vi "AlliGator Compute Lifetime Variance Map (Core).vi"(6 "Build New Maps":bool, 7 "Function Parameters":T1={"Function"=enum."Single-Exponential", "Amplitude"=0.0, "Exponent/Scale"=0.0, "Baseline"=0.0, "Residuals SDV"=0.0, "Minimum CL (%)"=1.0, "Analysis Type"=enum."Reference", "Bootstrap SDV x Scale Factor"=1.0, "Residuals SDV x Scale Factor"=1.0, "Low CL Percentile to Reject (%)"=1.0} {"Low CL Percentile to Reject (%)" min=0.0 max=100.0; "Residuals SDV x Scale Factor" min=0.0 max=100.0; "Bootstrap SDV x Scale Factor" min=0.0 max=100.0; "Minimum CL (%)" min=1.0}, 8 "error in (no error)":errorcluster, 11 "Lifetime Variance Data Array":T3[](array[typedef])) -> (0 "error out":errorcluster, 1 "CV Bootstrap SDV Test kappa x SDV":dbl, 2 "CV Residual Test kappa x SDV":dbl, 3 "Maps Data":dbl[][](array[numeric]))   [LabVIEW 2021, in "AlliGator Decay Fit Parameter Map.lvlib"]
uses:
  Decay Fit Parameter Map/AlliGator Decay Fit Parameter Map.lvlib
  Camera Noise Influence on Lifetime/Lifetime Variance Data.ctl
  Decay Fit Parameter Map/AlliGator Function Parameters.ctl
  Decay Fit Parameter Map/AlliGator CV(tau) Model Function.ctl
  Decay Fit Parameter Map/AlliGator Lifetime Variance Statistical Test.ctl
  <vilib>/gmath/statdist.llb/F CDF.vi
  <vilib>/gmath/statdist.llb/Normal CDF.vi
  <vilib>/gmath/statdist.llb/Normal Inverse CDF.vi
  <userlib>/_OpenG.lib/array/array.llb/Index 1D Array Elements (DBL)__ogtk.vi
  Error/Error.lvlib
  <vilib>/gmath/NI_Gmath.lvlib
  Arrays/Arrays.lvlib
  <userlib>/_OpenG.lib/array/array.llb/openg_array.lvlib
  Lifetime & Other Parameters/AlliGator Lifetime & Other Parameters.lvlib
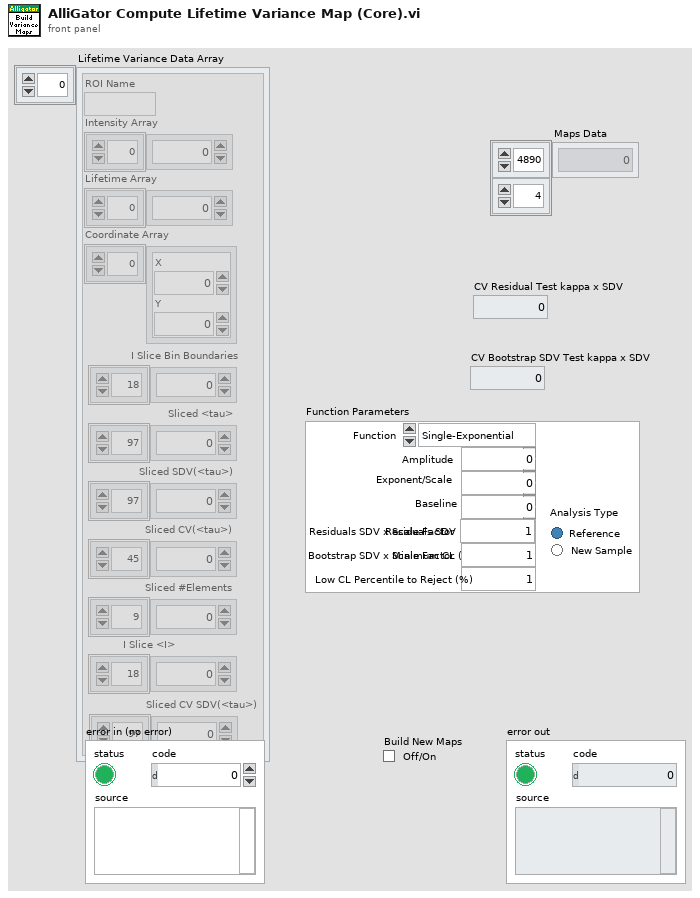
[diagram p1: front panel]
types:
  T1 = typedef "AlliGator Decay Fit Parameter Map.lvlib/AlliGator Function Parameters.ctl" = cluster{"Function":T2, "Amplitude":dbl, "Exponent/Scale":dbl, "Baseline":dbl, "Residuals SDV":dbl, "Minimum CL (%)":dbl, "Analysis Type":enum32{"Reference", "New Sample"}, "Bootstrap SDV x Scale Factor":dbl, "Residuals SDV x Scale Factor":dbl, "Low CL Percentile to Reject (%)":dbl}
  T2 = typedef "AlliGator Lifetime & Other Parameters.lvlib/AlliGator CV(tau) Model Function.ctl" = enum16{"Single-Exponential", "Power Law"}
  T3 = typedef "AlliGator Decay Fit Parameter Map.lvlib/Lifetime Variance Data.ctl" = cluster{"ROI Name":string, "Intensity Array":sgl[], "Lifetime Array":dbl[], "Coordinate Array":cluster{"X":i32, "Y":i32}[], "I Slice Bin Boundaries":dbl[], "Sliced <tau>":dbl[], "Sliced SDV(<tau>)":dbl[], "Sliced CV(<tau>)":dbl[], "Sliced #Elements":i32[], "I Slice <I>":dbl[], "Sliced CV SDV(<tau>)":dbl[]}
  T4 = typedef "AlliGator Decay Fit Parameter Map.lvlib/AlliGator Lifetime Variance Statistical Test.ctl" = enum16{"CV Approximate F-test", "Variance F-test", "CV Residuals test", "CV Bootstrap SDV Test"}
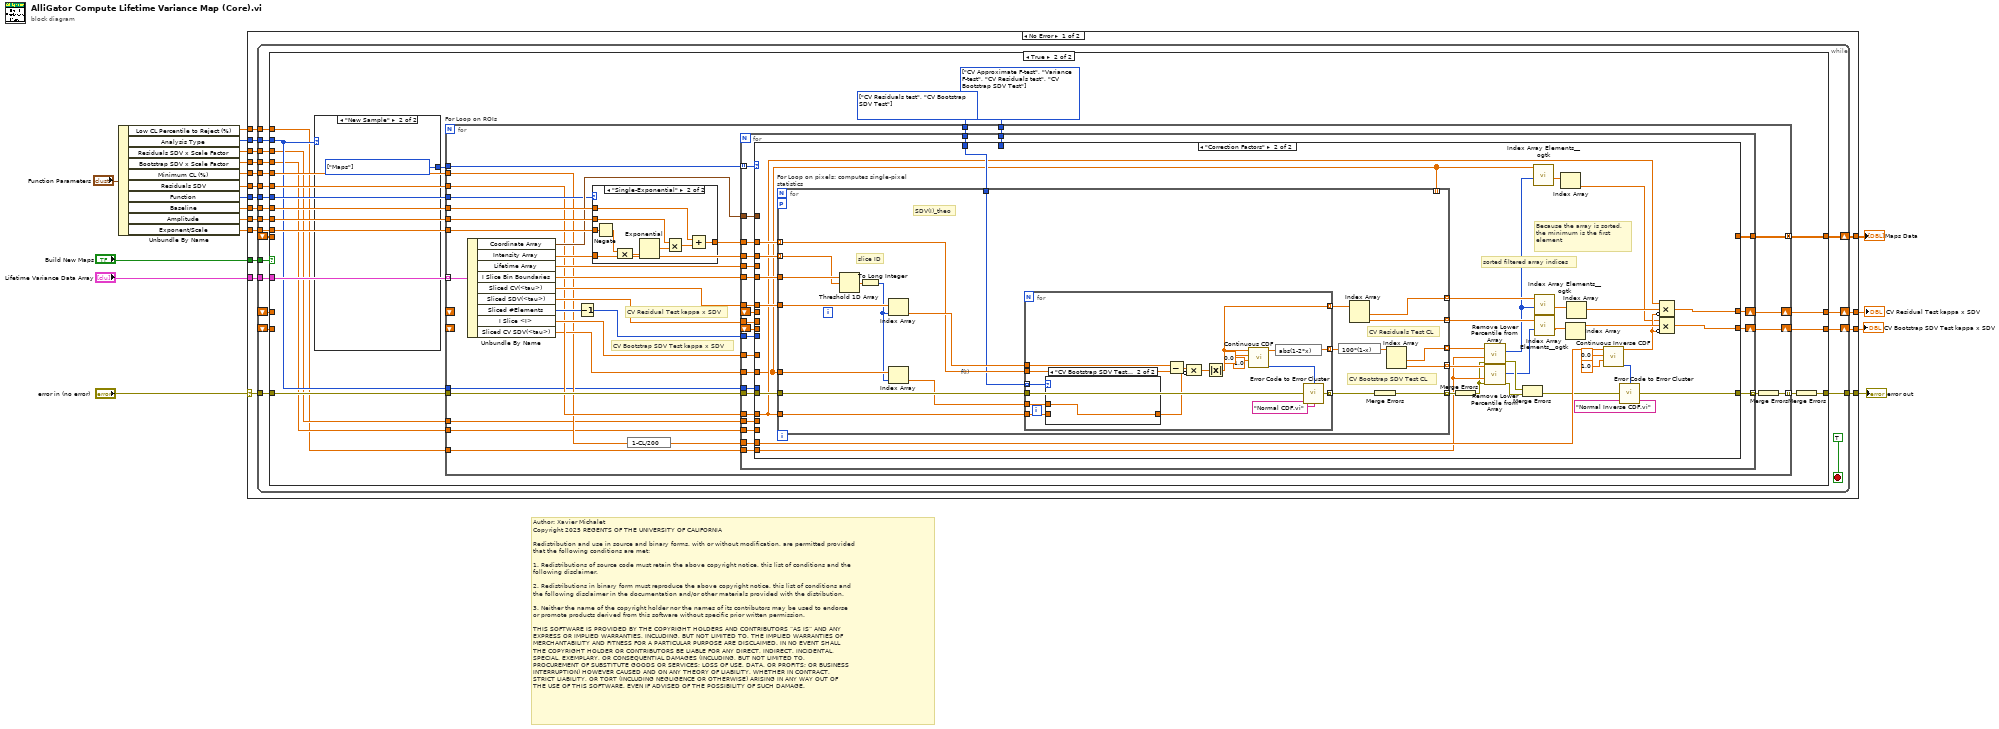
[diagram p0: block diagram]
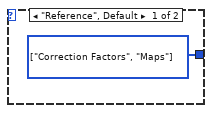
[diagram p3: hidden frame]
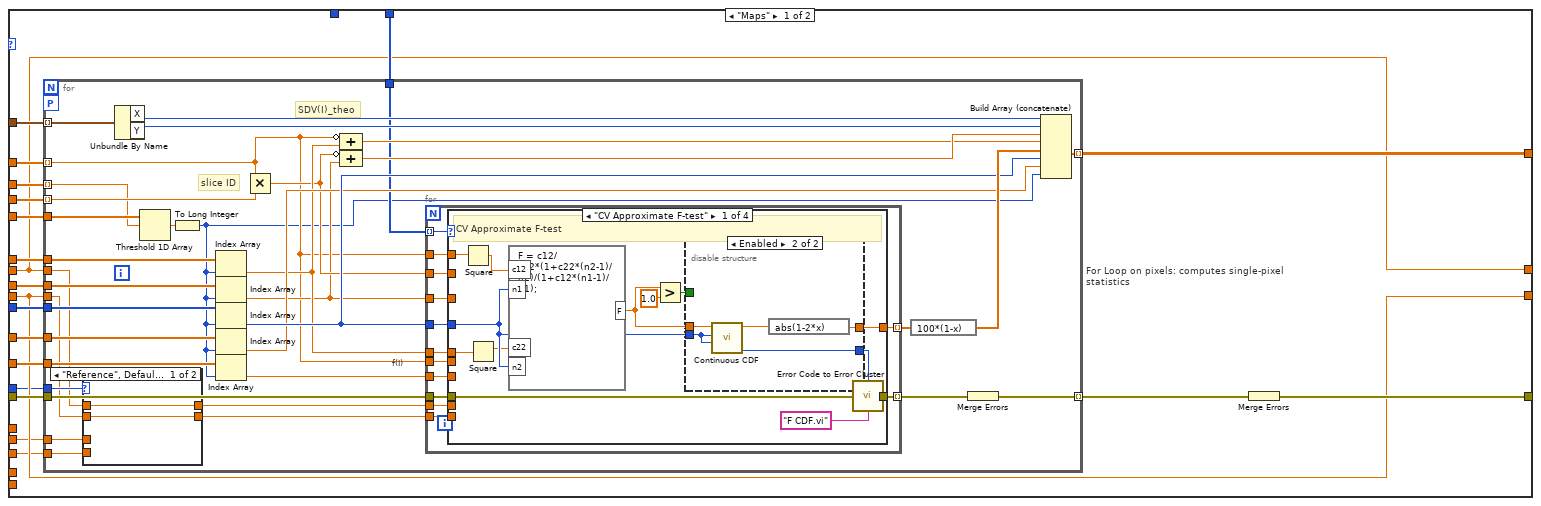
[diagram p4: hidden frame]
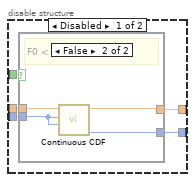
[diagram p6: hidden frame]
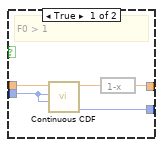
[diagram p7: hidden frame]
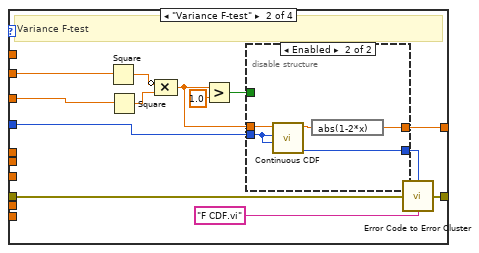
[diagram p8: hidden frame]
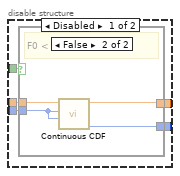
[diagram p9: hidden frame]
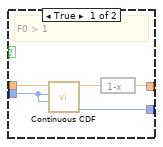
[diagram p10: hidden frame]
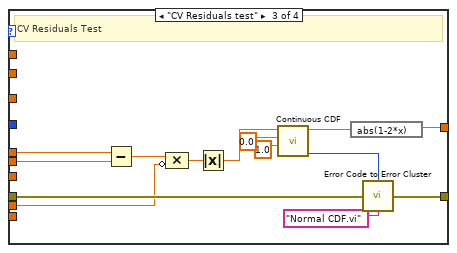
[diagram p11: hidden frame]
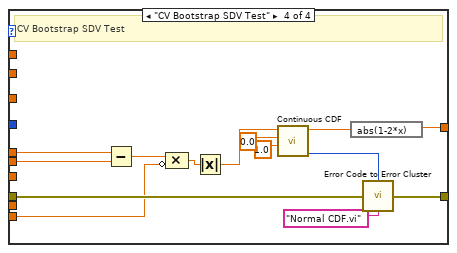
[diagram p12: hidden frame]
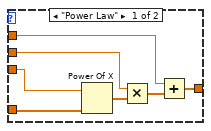
[diagram p14: hidden frame]
diagram:
  # "Author: Xavier Michalet\nCopyright 2025 REGENTS OF THE UNIVERSITY OF CALIFORNIA\n\nRedistribution and use in source and binary forms, with or without modification, are permitted provided\nthat the following conditions are met:\n\n1. Redistributions of source code must retain the above copyright notice, this list of conditions and the\nfollowing disclaimer.\n\n2. Redistributions in binary form must reproduce the above copyright notice, this list of conditions and\nthe following disclaimer in the documentation and/or other materials provided with the distribution.\n\n3. Neither the name of the copyright holder nor the names of its contributors may be used to endorse \nor promote products derived from this software without specific prior written permission.\n\nTHIS SOFTWARE IS PROVIDED BY THE COPYRIGHT HOLDERS AND CONTRIBUTORS “AS IS” AND ANY \nEXPRESS OR IMPLIED WARRANTIES, INCLUDING, BUT NOT LIMITED TO, THE IMPLIED WARRANTIES OF\nMERCHANTABILITY AND FITNESS FOR A PARTICULAR PURPOSE ARE DISCLAIMED. IN NO EVENT SHALL\nTHE COPYRIGHT HOLDER OR CONTRIBUTORS BE LIABLE FOR ANY DIRECT, INDIRECT, INCIDENTAL, \nSPECIAL, EXEMPLARY, OR CONSEQUENTIAL DAMAGES (INCLUDING, BUT NOT LIMITED TO, \nPROCUREMENT OF SUBSTITUTE GOODS OR SERVICES; LOSS OF USE, DATA, OR PROFITS; OR BUSINESS\nINTERRUPTION) HOWEVER CAUSED AND ON ANY THEORY OF LIABILITY, WHETHER IN CONTRACT, \nSTRICT LIABILITY, OR TORT (INCLUDING NEGLIGENCE OR OTHERWISE) ARISING IN ANY WAY OUT OF\nTHE USE OF THIS SOFTWARE, EVEN IF ADVISED OF THE POSSIBILITY OF SUCH DAMAGE."
  n1 = Unbundle By Name("Function Parameters") -> ("Low CL Percentile to Reject (%)"=w1:dbl, "Analysis Type"=w4:enum32{"Reference", "New Sample"}, "Residuals SDV x Scale Factor"=w3:dbl, "Bootstrap SDV x Scale Factor"=w2:dbl, "Minimum CL (%)"=w7:dbl, "Residuals SDV"=w8:dbl, "Function"=w9:T2, "Baseline"=w14:dbl, "Amplitude"=w15:dbl, "Exponent/Scale"=w16:dbl)
  n2 = case shown="No Error" "error in (no error)" {
    selector: "error in (no error)" -> [w28 w397]
    tunnel: "Lifetime Variance Data Array" -> [w35 _]
    tunnel: w16 -> [w34 _]
    tunnel: w15 -> [w33 _]
    tunnel: w14 -> [w32 _]
    tunnel: [w31 _] -> w13
    tunnel: "Build New Maps" -> [w30 _]
    tunnel: [w29 w397] -> w10
    tunnel: w9 -> [w27 _]
    tunnel: w8 -> [w26 _]
    tunnel: w7 -> [w25 _]
    tunnel: [w24 _] -> w6
    tunnel: [w23 _] -> w5
    tunnel: w4 -> [w22 _]
    tunnel: w3 -> [w21 _]
    tunnel: w2 -> [w20 _]
    tunnel: w1 -> [w19 _]
    frame No Error {
      n3 = while {
        tunnel: w35 -> [w56]
        tunnel: w34 -> [w55]
        tunnel: w33 -> [w54]
        tunnel: w32 -> [w53]
        tunnel: w30 -> [w51]
        shift-right: [w52] -> w31
        shift-left: _ -> [w49]
        tunnel: [w48] -> w29
        tunnel: w28 -> [w47]
        tunnel: w27 -> [w46]
        tunnel: w26 -> [w45]
        tunnel: w25 -> [w44]
        shift-right: [w43] -> w24
        shift-left: _ -> [w41]
        shift-right: [w42] -> w23
        shift-left: _ -> [w40]
        tunnel: w22 -> [w39]
        tunnel: w21 -> [w38]
        tunnel: w20 -> [w37]
        tunnel: w19 -> [w36]
        stop <- TRUE stop-if-true
        n4 = case shown="True" w51 {
          tunnel: w56 -> [_ w80]
          tunnel: w55 -> [_ w79]
          tunnel: w54 -> [_ w78]
          tunnel: w53 -> [_ w77]
          tunnel: [w60 w76] -> w52
          tunnel: w49 -> [w60 _]
          tunnel: [w59 w74] -> w48
          tunnel: w47 -> [w59 w73]
          tunnel: w46 -> [_ w72]
          tunnel: w45 -> [_ w71]
          tunnel: w44 -> [_ w69]
          tunnel: [w58 w67] -> w43
          tunnel: [w57 w66] -> w42
          tunnel: w41 -> [w58 _]
          tunnel: w40 -> [w57 _]
          tunnel: w39 -> [_ w64]
          tunnel: w38 -> [_ w63]
          tunnel: w37 -> [_ w62]
          tunnel: w36 -> [_ w61]
          frame False {
          }
          frame True {
            w68 = T4[] [enum."CV Residuals test", enum."CV Bootstrap SDV Test"] items=["CV Approximate F-test", "Variance F-test", "CV Residuals test", "CV Bootstrap SDV Test"]
            w70 = T4[] [enum."CV Approximate F-test", enum."Variance F-test", enum."CV Residuals test", enum."CV Bootstrap SDV Test"] items=["CV Approximate F-test", "Variance F-test", "CV Residuals test", "CV Bootstrap SDV Test"]
            n5 = case shown="\"New Sample\"" w64 {
              tunnel: [w81 w82] -> w65
              frame "Reference", Default {
                w81 = enum16{"Correction Factors", "Maps"}[] [enum."Correction Factors", enum."Maps"] items=["Correction Factors", "Maps"]
              }
              frame "New Sample" {
                w82 = enum16{"Correction Factors", "Maps"}[] [enum."Maps"] items=["Correction Factors", "Maps"]
              }
            }
            n6 = for "For Loop on ROIs" {
              tunnel: w80 -> [w114] mode=indexing
              tunnel: w79 -> [w113]
              tunnel: w78 -> [w112]
              tunnel: w77 -> [w111]
              tunnel: [w101] -> w76 mode=concatenating
              tunnel: [w99] -> w75 mode=indexing
              tunnel: w73 -> [w98]
              tunnel: w72 -> [w96]
              tunnel: w71 -> [w95]
              tunnel: w70 -> [w94]
              tunnel: w69 -> [w91]
              tunnel: w65 -> [w92]
              tunnel: w68 -> [w89]
              shift-right: [w88] -> w67
              shift-left: _ -> [_]
              shift-right: [w87] -> w66
              shift-left: _ -> [_]
              tunnel: w64 -> [w86]
              tunnel: w63 -> [w85]
              tunnel: w62 -> [w84]
              tunnel: w61 -> [w83]
              # "CV Bootstrap SDV Test kappa x SDV"
              # "CV Residual Test kappa x SDV"
              n7 = Unbundle By Name(w114) -> ("Coordinate Array"=w105:cluster{"X":i32, "Y":i32}[], "Intensity Array"=w104:sgl[], "Lifetime Array"=w110:dbl[], "I Slice Bin Boundaries"=w109:dbl[], "Sliced CV(<tau>)"=w108:dbl[], "Sliced SDV(<tau>)"=w106:dbl[], "Sliced #Elements"=w103:i32[], "I Slice <I>"=w97:dbl[], "Sliced CV SDV(<tau>)"=w93:dbl[])
              n8 = Decrement(x=w103) -> (x-1=w102:i32[])
              n9 = case shown="\"Single-Exponential\"" w96 {
                tunnel: w113 -> [w387 w389]
                tunnel: w112 -> [w385 w395]
                tunnel: w111 -> [w383 w393]
                tunnel: [w382 w392] -> w107
                tunnel: w104 -> [w381 w391]
                frame "Power Law" {
                  n10 = Power Of X(1:w381, 2:w387) -> (0:w386:dbl[])
                  n11 = Multiply(x=w385, y=w386) -> (x*y=w384:dbl[])
                  n12 = Add(x=w383, y=w384) -> (x+y=w382:dbl[])
                }
                frame "Single-Exponential" {
                  n13 = Negate(x=w389) -> (-x=w388:dbl)
                  n14 = Compound Arithmetic op=MULTIPLY(w388, w391) -> (w390:dbl[])
                  n15 = Exponential(1:w390) -> (0:w396:dbl[])
                  n16 = Multiply(x=w395, y=w396) -> (x*y=w394:dbl[])
                  n17 = Add(x=w393, y=w394) -> (x+y=w392:dbl[])
                }
              }
              n18 = expression code="1-CL/200"(w91) -> (w90:dbl)
              n19 = for {
                tunnel: w110 -> [w140]
                tunnel: w109 -> [w139]
                tunnel: w108 -> [w138]
                tunnel: w107 -> [w137]
                tunnel: w106 -> [w136]
                tunnel: w105 -> [w135]
                tunnel: w104 -> [w134]
                tunnel: w102 -> [w133]
                tunnel: [w132] -> w101
                tunnel: [w131] -> w100 mode=indexing
                tunnel: w98 -> [w130]
                tunnel: w97 -> [w129]
                tunnel: w95 -> [w128]
                tunnel: w94 -> [w127]
                tunnel: w93 -> [w126]
                tunnel: w90 -> [w125]
                tunnel: w92 -> [w124] mode=indexing
                shift-right: [w123] -> w88
                shift-left: _ -> [w121]
                shift-right: [w122] -> w87
                shift-left: _ -> [w120]
                tunnel: w89 -> [w119]
                tunnel: w86 -> [w118]
                tunnel: w85 -> [w117]
                tunnel: w84 -> [w116]
                tunnel: w83 -> [w115]
                n20 = case shown="\"Correction Factors\"" w124 {
                  tunnel: w140 -> [w160 _]
                  tunnel: w139 -> [w159 w340]
                  tunnel: w138 -> [w158 w339]
                  tunnel: w137 -> [w157 w338]
                  tunnel: w136 -> [w156 _]
                  tunnel: w135 -> [w155 _]
                  tunnel: w134 -> [w154 w337]
                  tunnel: w133 -> [w153 _]
                  tunnel: [w152 _] -> w132
                  tunnel: [w146 w328] -> w131
                  tunnel: w130 -> [w150 w335]
                  tunnel: w129 -> [w149 _]
                  tunnel: w128 -> [_ w310]
                  tunnel: w127 -> [w148 _]
                  tunnel: w126 -> [w147 w309]
                  tunnel: w125 -> [_ w325]
                  tunnel: [w145 w327] -> w123
                  tunnel: [w144 w326] -> w122
                  tunnel: w121 -> [w145 _]
                  tunnel: w120 -> [w144 _]
                  tunnel: w119 -> [_ w323]
                  tunnel: w118 -> [w143 _]
                  tunnel: w117 -> [w142 _]
                  tunnel: w116 -> [w141 _]
                  tunnel: w115 -> [_ w320]
                  frame "Maps" {
                    n21 = for "For Loop on pixels: computes single-pixel statistics" {
                      tunnel: w160 -> [w193] mode=indexing
                      tunnel: w159 -> [w196]
                      tunnel: w158 -> [w195]
                      tunnel: w157 -> [w172] mode=indexing
                      tunnel: w156 -> [w194]
                      tunnel: w155 -> [w192] mode=indexing
                      tunnel: w154 -> [w191] mode=indexing
                      tunnel: w153 -> [w186]
                      tunnel: [w183] -> w152 mode=indexing
                      tunnel: [w177] -> w151 mode=indexing
                      tunnel: w150 -> [w181]
                      tunnel: w149 -> [w180]
                      tunnel: w148 -> [w173]
                      tunnel: w147 -> [w171]
                      workers-P: _ -> [_]
                      tunnel: w145 -> [w166]
                      tunnel: w144 -> [w165]
                      tunnel: w143 -> [w167]
                      tunnel: w142 -> [w162]
                      tunnel: w141 -> [w161]
                      # "f(I)"
                      # "slice ID"
                      # "SDV(I)_theo"
                      n22 = case shown="\"Reference\", Default" w167 {
                        tunnel: w166 -> [w198 _]
                        tunnel: w165 -> [w197 _]
                        tunnel: [w198 w200] -> w164
                        tunnel: [w197 w199] -> w163
                        tunnel: w162 -> [_ w200]
                        tunnel: w161 -> [_ w199]
                        frame "Reference", Default {
                        }
                        frame "New Sample" {
                        }
                      }
                      n23 = Unbundle By Name(w192) -> ("X"=w190:i32, "Y"=w189:i32)
                      n24 = Threshold 1D Array(2:w191, 3:w196) -> (0:w170:dbl)  [unwired: 1 in]
                      n25 = To Long Integer(number=w170) -> (32bit integer=w168:i32)
                      n26 = Index Array(array=w195, index=w168) -> (element=w176:dbl)
                      n27 = Index Array(array=w194, index=w168) -> (element=w174:dbl)
                      n28 = Index Array(array=w186, index=w168) -> (element=w179:i32)
                      n29 = Index Array(array=w180, index=w168) -> (element=w178:dbl)
                      n30 = Index Array(array=w171, index=w168) -> (element=w169:dbl)
                      n31 = Multiply(x=w172, y=w193) -> (x*y=w175:dbl)
                      n32 = Compound Arithmetic op=ADD(invert w172, w176) -> (w187:dbl)
                      n33 = Compound Arithmetic op=ADD(invert w175, w174) -> (w188:dbl)
                      n34 = for {
                        tunnel: w179 -> [w210]
                        tunnel: w173 -> [w209] mode=indexing
                        tunnel: [w213] -> w185 mode=indexing
                        tunnel: w181 -> [w211]
                        tunnel: [w212] -> w182 mode=indexing
                        tunnel: w172 -> [w208]
                        tunnel: w176 -> [w207]
                        tunnel: w175 -> [w206]
                        tunnel: w174 -> [w205]
                        tunnel: w172 -> [w204]
                        tunnel: w169 -> [w203]
                        tunnel: w164 -> [w202]
                        tunnel: w163 -> [w201]
                        n35 = case shown="\"CV Approximate F-test\"" w209 {
                          tunnel: [w226 w258 w291 w305] -> w213
                          tunnel: [w225 w257 w290 w304] -> w212
                          tunnel: w211 -> [w222 w254 w287 w301]
                          tunnel: w210 -> [w216 w253 _ _]
                          tunnel: w208 -> [_ _ w284 w298]
                          tunnel: w207 -> [w218 _ w285 w299]
                          tunnel: w206 -> [_ w250 _ _]
                          tunnel: w205 -> [_ w249 _ _]
                          tunnel: w204 -> [w219 _ _ _]
                          tunnel: w203 -> [_ _ _ _]
                          tunnel: w202 -> [_ _ w278 _]
                          tunnel: w201 -> [_ _ _ w292]
                          frame "CV Approximate F-test" {
                            # "CV Approximate F-test"
                            n36 = Square(x=w219) -> (x^2=w217:dbl)
                            n37 = Square(x=w218) -> (x^2=w215:dbl)
                            n38 = formula code="F = c12/c22*(1+c22*(n2-1)/n2)/(1+c12*(n1-1)/n1);"("c12"=w217, "c22"=w215, "n1"=w216, "n2"=w216) -> ("F"=w214:dbl)
                            n39 = Greater?(x=w214, y=1.0) -> (0:w220:bool)
                            n40 = disable-structure shown="Enabled" {
                              disable-tunnel: [w231 w241] -> w226
                              disable-tunnel: [w230 w245] -> w224
                              disable-tunnel: w216 -> [w229 w244]
                              disable-tunnel: w214 -> [w228 w243]
                              disable-tunnel: w220 -> [w227 _]
                              frame Disabled {
                                n41 = case shown="False" w227 {
                                tunnel: w228 -> [w236 w240]
                                tunnel: [w232 w237] -> w231
                                tunnel: [w235 w239] -> w230
                                tunnel: w229 -> [w234 w238]
                                frame True {
                                # "F0 > 1"
                                n42 = call-poly <vilib>:"Continuous CDF.vi"("k2"=w234, "k1"=w234, "x"=w236) -> ("error"=w235:i32, "cdf(x)"=w233:dbl)  [unwired: 7 in]
                                n43 = expression code="1-x"(w233) -> (w232:dbl)
                                }
                                frame False {
                                # "F0 < 1"
                                n44 = call-poly <vilib>:"Continuous CDF.vi"("k2"=w238, "k1"=w238, "x"=w240) -> ("error"=w239:i32, "cdf(x)"=w237:dbl)  [unwired: 7 in]
                                }
                                }
                              }
                              frame Enabled {
                                n45 = call-poly <vilib>:"Continuous CDF.vi"("k2"=w244, "k1"=w244, "x"=w243) -> ("error"=w245:i32, "cdf(x)"=w242:dbl)  [unwired: 7 in]
                                n46 = expression code="abs(1-2*x)"(w242) -> (w241:dbl)
                              }
                            }
                            n47 = call "Error Code to Error Cluster.vi"("Error Code"=w224, "Error Source"="F CDF.vi", "Error In"=w222) -> ("Error Out"=w225:errorcluster)  [unwired: 12 in]
                          }
                          frame "Variance F-test" {
                            # "Variance F-test"
                            n48 = Square(x=w250) -> (x^2=w248:dbl)
                            n49 = Square(x=w249) -> (x^2=w251:dbl)
                            n50 = Compound Arithmetic op=MULTIPLY(invert w248, w251) -> (w247:dbl)
                            n51 = Greater?(x=w247, y=1.0) -> (0:w246:bool)
                            n52 = disable-structure shown="Enabled" {
                              disable-tunnel: [w263 w273] -> w258
                              disable-tunnel: [w262 w277] -> w256
                              disable-tunnel: w253 -> [w261 w276]
                              disable-tunnel: w247 -> [w260 w275]
                              disable-tunnel: w246 -> [w259 _]
                              frame Disabled {
                                n53 = case shown="False" w259 {
                                tunnel: w260 -> [w268 w272]
                                tunnel: [w264 w269] -> w263
                                tunnel: [w267 w271] -> w262
                                tunnel: w261 -> [w266 w270]
                                frame True {
                                # "F0 > 1"
                                n54 = call-poly <vilib>:"Continuous CDF.vi"("k2"=w266, "k1"=w266, "x"=w268) -> ("error"=w267:i32, "cdf(x)"=w265:dbl)  [unwired: 7 in]
                                n55 = expression code="1-x"(w265) -> (w264:dbl)
                                }
                                frame False {
                                # "F0 < 1"
                                n56 = call-poly <vilib>:"Continuous CDF.vi"("k2"=w270, "k1"=w270, "x"=w272) -> ("error"=w271:i32, "cdf(x)"=w269:dbl)  [unwired: 7 in]
                                }
                                }
                              }
                              frame Enabled {
                                n57 = call-poly <vilib>:"Continuous CDF.vi"("k2"=w276, "k1"=w276, "x"=w275) -> ("error"=w277:i32, "cdf(x)"=w274:dbl)  [unwired: 7 in]
                                n58 = expression code="abs(1-2*x)"(w274) -> (w273:dbl)
                              }
                            }
                            n59 = call "Error Code to Error Cluster.vi"("Error Code"=w256, "Error Source"="F CDF.vi", "Error In"=w254) -> ("Error Out"=w257:errorcluster)  [unwired: 12 in]
                          }
                          frame "CV Residuals test" {
                            # "CV Residuals Test"
                            n60 = Subtract(x=w285, y=w284) -> (x-y=w283:dbl)
                            n61 = Compound Arithmetic op=MULTIPLY(w283, invert w278) -> (w282:dbl)
                            n62 = Absolute Value(x=w282) -> (abs(x)=w279:dbl)
                            n63 = call-poly <vilib>:"Continuous CDF.vi"("std"=1.0, "mean"=0.0, "x"=w279) -> ("error"=w289:i32, "cdf(x)"=w286:dbl)  [unwired: 7 in]
                            n64 = expression code="abs(1-2*x)"(w286) -> (w291:dbl)
                            n65 = call "Error Code to Error Cluster.vi"("Error Code"=w289, "Error Source"="Normal CDF.vi", "Error In"=w287) -> ("Error Out"=w290:errorcluster)  [unwired: 12 in]
                          }
                          frame "CV Bootstrap SDV Test" {
                            # "CV Bootstrap SDV Test"
                            n66 = Subtract(x=w299, y=w298) -> (x-y=w297:dbl)
                            n67 = Compound Arithmetic op=MULTIPLY(w297, invert w292) -> (w296:dbl)
                            n68 = Absolute Value(x=w296) -> (abs(x)=w293:dbl)
                            n69 = call-poly <vilib>:"Continuous CDF.vi"("std"=1.0, "mean"=0.0, "x"=w293) -> ("error"=w303:i32, "cdf(x)"=w300:dbl)  [unwired: 7 in]
                            n70 = expression code="abs(1-2*x)"(w300) -> (w305:dbl)
                            n71 = call "Error Code to Error Cluster.vi"("Error Code"=w303, "Error Source"="Normal CDF.vi", "Error In"=w301) -> ("Error Out"=w304:errorcluster)  [unwired: 12 in]
                          }
                        }
                      }
                      n72 = expression code="100*(1-x)"(w185) -> (w184:dbl[])
                      n73 = Merge Errors(w182) -> (w177:errorcluster)
                      n74 = Build Array (concatenate)(w190, w189, w188, w187, w184, w179, w178, w168) -> (w183:dbl[])
                    }
                    n75 = Merge Errors(w151) -> (w146:errorcluster)
                  }
                  frame "Correction Factors" {
                    # "Because the array is sorted, the minimum is the first element"
                    # "sorted filtered array indices"
                    n76 = for "For Loop on pixels: computes single-pixel statistics" {
                      tunnel: w340 -> [w361]
                      tunnel: w339 -> [w360]
                      tunnel: w338 -> [w352] mode=indexing
                      tunnel: w337 -> [w359] mode=indexing
                      tunnel: [w355] -> w336 mode=indexing
                      tunnel: w335 -> [w356]
                      tunnel: w310 -> [w354]
                      tunnel: w309 -> [w351]
                      workers-P: _ -> [_]
                      tunnel: [w346] -> w322 mode=indexing
                      tunnel: [w345] -> w321 mode=indexing
                      tunnel: [w343] -> w315 mode=indexing
                      tunnel: [w342] -> w313 mode=indexing
                      tunnel: w323 -> [w341]
                      tunnel: w309 -> [_] mode=indexing
                      # "CV Bootstrap SDV Test CL"
                      # "CV Residuals Test CL"
                      # "f(I)"
                      # "slice ID"
                      # "SDV(I)_theo"
                      n77 = Threshold 1D Array(2:w359, 3:w361) -> (0:w350:dbl)  [unwired: 1 in]
                      n78 = To Long Integer(number=w350) -> (32bit integer=w348:i32)
                      n79 = Index Array(array=w360, index=w348) -> (element=w353:dbl)
                      n80 = Index Array(array=w351, index=w348) -> (element=w349:dbl)
                      n81 = for {
                        tunnel: w341 -> [w365] mode=indexing
                        tunnel: [w378] -> w358 mode=indexing
                        tunnel: w356 -> [w376]
                        tunnel: [w377] -> w357 mode=indexing
                        tunnel: w354 -> [w363]
                        tunnel: w352 -> [w375]
                        tunnel: w353 -> [w374]
                        tunnel: w349 -> [w364]
                        tunnel: [w373] -> w344 mode=indexing
                        n82 = case shown="\"CV Bootstrap SDV Test\"" w365 {
                          tunnel: w364 -> [_ w380]
                          tunnel: w363 -> [w379 _]
                          tunnel: [w379 w380] -> w362
                          frame "CV Residuals test", Default {
                          }
                          frame "CV Bootstrap SDV Test" {
                          }
                        }
                        n83 = Subtract(x=w374, y=w375) -> (x-y=w369:dbl)
                        n84 = Compound Arithmetic op=MULTIPLY(w369, invert w362) -> (w368:dbl)
                        n85 = Absolute Value(x=w368) -> (abs(x)=w373:dbl)
                        n86 = call-poly <vilib>:"Continuous CDF.vi"("std"=1.0, "mean"=0.0, "x"=w373) -> ("error"=w372:i32, "cdf(x)"=w370:dbl)  [unwired: 7 in]
                        n87 = expression code="abs(1-2*x)"(w370) -> (w378:dbl)
                        n88 = call "Error Code to Error Cluster.vi"("Error Code"=w372, "Error Source"="Normal CDF.vi", "Error In"=w376) -> ("Error Out"=w377:errorcluster)  [unwired: 12 in]
                      }
                      n89 = expression code="100*(1-x)"(w358) -> (w347:dbl[])
                      n90 = Index Array(array=w344) -> (element #1=w343:dbl, element #2=w342:dbl)  [unwired: 2 in]
                      n91 = Merge Errors(w357) -> (w355:errorcluster)
                      n92 = Index Array(array=w347) -> (element #1=w346:dbl, element #2=w345:dbl)  [unwired: 2 in]
                    }
                    n93 = Merge Errors(w336) -> (w319:errorcluster)
                    n94 = call "Remove Lower Percentile from Array.vi"("Error In"=w319, "Low Percentile to Reject"=w320, "Array in"=w322) -> ("Error Out"=w316:errorcluster, "Array Indices out"=w308:i32[])  [unwired: 5 in, 2 out]
                    n95 = call "Remove Lower Percentile from Array.vi"("Error In"=w319, "Low Percentile to Reject"=w320, "Array in"=w321) -> ("Error Out"=w318:errorcluster, "Array Indices out"=w312:i32[])  [unwired: 5 in, 2 out]
                    n96 = Merge Errors(w316, w318) -> (w317:errorcluster)
                    n97 = call-poly <userlib>:"Index Array Elements__ogtk.vi"("indices"=w308, "array"=w309) -> ("elements"=w307:dbl[])  [unwired: 9 in]
                    n98 = call-poly <userlib>:"Index Array Elements__ogtk.vi"("indices"=w308, "array"=w315) -> ("elements"=w314:dbl[])  [unwired: 9 in]
                    n99 = call-poly <userlib>:"Index Array Elements__ogtk.vi"("indices"=w312, "array"=w313) -> ("elements"=w311:dbl[])  [unwired: 9 in]
                    n100 = Index Array(array=w307) -> (element=w306:dbl)  [unwired: 1 in]
                    n101 = Index Array(array=w311) -> (element=w331:dbl)  [unwired: 1 in]
                    n102 = Index Array(array=w314) -> (element=w332:dbl)  [unwired: 1 in]
                    n103 = call-poly <vilib>:"Continuous Inverse CDF.vi"("std"=1.0, "mean"=0.0, "cdf(x)"=w325) -> ("error"=w329:i32, "x"=w324:dbl)  [unwired: 7 in]
                    n104 = call "Error Code to Error Cluster.vi"("Error Code"=w329, "Error Source"="Normal Inverse CDF.vi", "Error In"=w317) -> ("Error Out"=w328:errorcluster)  [unwired: 12 in]
                    n105 = Compound Arithmetic op=MULTIPLY(w310, w332, invert w324) -> (w327:dbl)
                    n106 = Compound Arithmetic op=MULTIPLY(w306, w331, invert w324) -> (w326:dbl)
                  }
                }
              }
              n107 = Merge Errors(w100) -> (w99:errorcluster)
            }
            n108 = Merge Errors(w75) -> (w74:errorcluster)
          }
        }
      }
    }
    frame Error {
    }
  }
  "error out" <- w10
  "Maps Data" <- w13
  "CV Residual Test kappa x SDV" <- w6
  "CV Bootstrap SDV Test kappa x SDV" <- w5
